vi "Servo MoveBy.vi"(8 "error in":errorcluster, 10 "Move by":dbl, 11 "Status in":T1={"Servo variables"={"Terget reached"=FALSE, "Connected"=FALSE, "Power ON"=FALSE, "Operation mode"=FALSE, "Actual position"=0.0, "Target position"=0.0}, "Servo constants"={"Name"=enum."AxisX", "Pos position limit [mm]"=0.0, "Neg position limit [mm]"=0.0, "Pos velocity limit"=0.0, "Neg velocity limit"=0.0, "Acceleration limit"=0.0}, "Connection"=variant}) -> (0 "error out":errorcluster, 1 "executed":bool, 2 "Target position":dbl, 3 "connection out":variant)   [LabVIEW 2024, in "Servo drive module.lvlib"]
doc: "Executes an additive move from an actual position to a desired position.\nParams:\nStatus in - actual status of servo drive.\nMove by - a numeric of desired change of position for servo drive.\nReturns: \nTrget position\nExecuted - True, if execution was sucessful."
uses:
  Servo drive module.lvlib
  ctl/Servo state.ctl
  ctl/Servo variables.ctl
  ctl/Servo constants.ctl
  ctl/Axis names.ctl
  <vilib>/Utility/error.llb/Error Cluster From Error Code.vi
  <vilib>/ErrorRing/Error Ring.xnode
  <vilib>/addons/eal4LabVIEW/eal4LabVIEW.lvlib
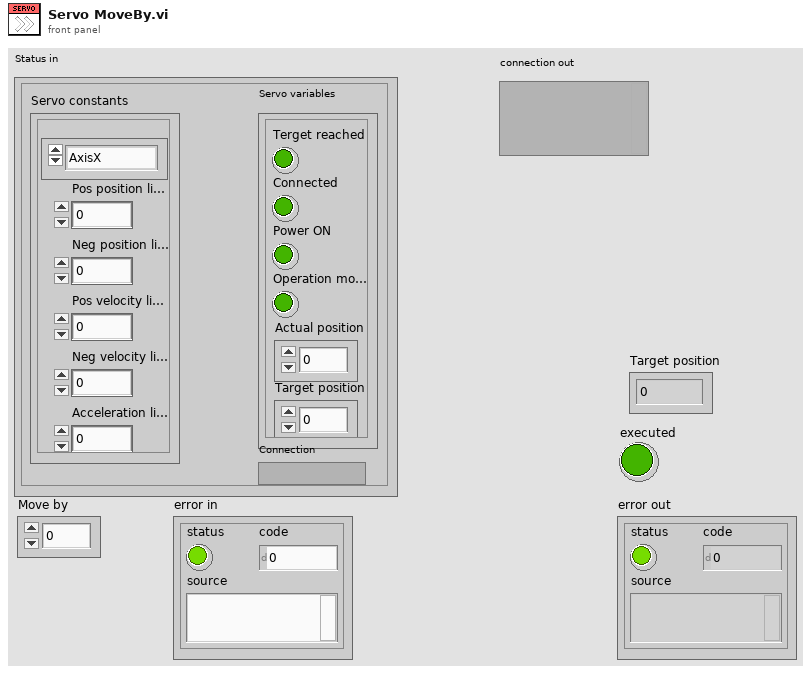
[diagram p1: front panel]
types:
  T1 = typedef "Servo drive module.lvlib/Servo state.ctl" = cluster{"Servo variables":T2, "Servo constants":T3, "Connection":variant}
  T2 = typedef "Servo drive module.lvlib/Servo variables.ctl" = cluster{"Terget reached":bool, "Connected":bool, "Power ON":bool, "Operation mode":bool, "Actual position":dbl, "Target position":dbl}
  T3 = typedef "Servo drive module.lvlib/Servo constants.ctl" = cluster{"Name":T4, "Pos position limit [mm]":dbl, "Neg position limit [mm]":dbl, "Pos velocity limit":dbl, "Neg velocity limit":dbl, "Acceleration limit":dbl}
  T4 = typedef "Servo drive module.lvlib/Axis names.ctl" = enum16{"Unknown", "AxisX", "AxisY", "AxisZ_left", "AxisZ_middle", "AxisZ_right"}
  T5 = cluster{"Position":dbl, "Velocity":dbl, "Acceleration":dbl, "Deceleration":dbl, "Jerk":dbl}
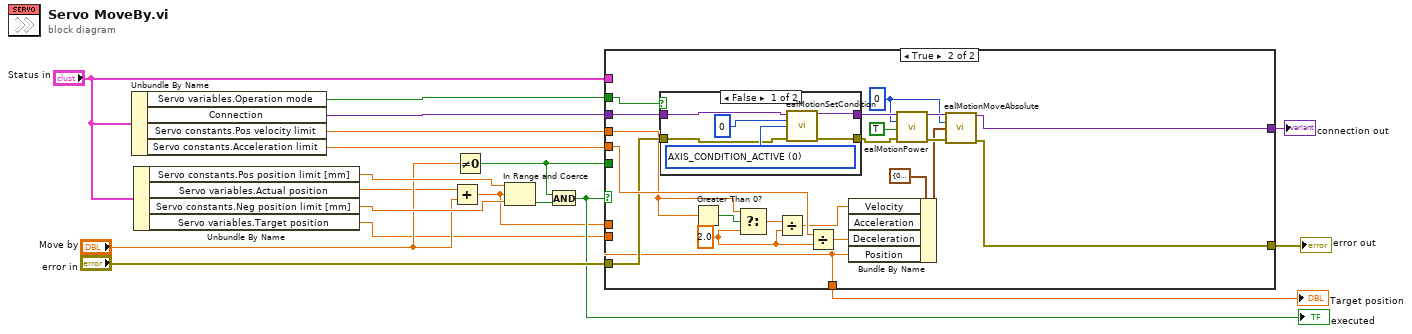
[diagram p0: block diagram]
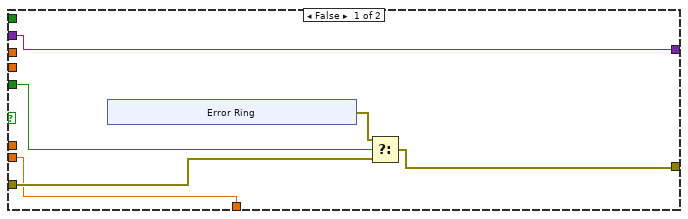
[diagram p2: hidden frame]
diagram:
  n1 = Unbundle By Name("Status in") -> ("Servo variables.Operation mode"=w16:bool, "Connection"=w15:variant, "Servo constants.Pos velocity limit"=w10:dbl, "Servo constants.Acceleration limit"=w9:dbl)
  n2 = Unbundle By Name("Status in") -> ("Servo constants.Pos position limit [mm]"=w14:dbl, "Servo variables.Actual position"=w2:dbl, "Servo constants.Neg position limit [mm]"=w13:dbl, "Servo variables.Target position"=w1:dbl)
  n3 = Add(x=w2, y="Move by") -> (x+y=w4:dbl)
  n4 = Not Equal To 0?(x="Move by") -> (x != 0?=w7:bool)
  n5 = In Range and Coerce(upper limit=w14, x=w4, lower limit=w13) -> (In Range?=w8:bool)  [unwired: 1 out]
  n6 = And(x=w7, y=w8) -> (x .and. y?=w5:bool)
  "executed" <- w5
  n7 = case shown="True" w5 {
    tunnel: w4 -> [_ w29]
    tunnel: [w24 w33] -> w18
    tunnel: "error in" -> [w22 w38]
    tunnel: "Status in" -> [_ _]
    tunnel: w15 -> [w20 w49]
    tunnel: w10 -> [_ w36]
    tunnel: w9 -> [_ w48]
    tunnel: w16 -> [_ w39]
    tunnel: w7 -> [w23 _]
    tunnel: [w20 w32] -> w6
    tunnel: [w19 w29] -> w3
    tunnel: w1 -> [w19 _]
    frame False {
      n8 = xnode "Error Ring"() -> ("error out"=w21:errorcluster)
      n9 = Select(t=w21, s=w23, f=w22) -> (s? t:f=w24:errorcluster)
    }
    frame True {
      w40 = 0 ("slave index")
      w34 = 2.0 ("y")
      n10 = case shown="False" w39 {
        tunnel: [w55 w57] -> w43
        tunnel: [w53 w56] -> w44
        tunnel: w49 -> [w52 w57]
        tunnel: w38 -> [w50 w56]
        frame False {
          w54 = 0 items=["AXIS_CONDITION_ACTIVE"=0, "AXIS_CONDITION_PARKING"=1, "AXIS_CONDITION_DEACTIVATED"=2, "AXIS_CONDITION_ACTIVE_DECOUPLED"=4, "AXIS_CONDITION_PARKING_DECOUPLED"=5, "AXIS_CONDITION_DEACTIVATED_DECOUPLED"=6, "AXIS_CONDITION_ACTIVE_PARAMETERIZATION"=8, "AXIS_CONDITION_PARKING_PARAMETERIZATION"=9, "AXIS_CONDITION_DEACTIVATED_PARAMETERIZATION"=10, "AXIS_CONDITION_ACTIVE_DECOUPLED_PARAMETERIZATION"=12, "AXIS_CONDITION_PARKING_DECOUPLED_PARAMETERIZATION"=13, "AXIS_CONDITION_DEACTIVATED_DECOUPLED_PARAMETERIZATION"=14] ("condition")
          n11 = call <vilib>:"ealMotionSetCondition.vi"("connection in"=w52, "slave index"=0, "condition"=w54, "error in (no error)"=w50) -> ("connection out"=w55:variant, "error out"=w53:errorcluster)  [unwired: 10 in]
        }
        frame True {
        }
      }
      n12 = Greater Than 0?(x=w36) -> (x > 0?=w37:bool)
      n13 = Select(t=w36, s=w37, f=w34) -> (s? t:f=w35:dbl)
      n14 = Divide(x=w35, y=w34) -> (x/y=w42:dbl)
      n15 = Divide(x=w48, y=w34) -> (x/y=w41:dbl)
      n16 = Bundle By Name(cluster=T5 {"Position"=0.0, "Velocity"=500.0, "Acceleration"=500.0, "Deceleration"=500.0, "Jerk"=500.0} ("parameter set"), "Velocity"=w42, "Acceleration"=w41, "Deceleration"=w41, "Position"=w29) -> (w31:T5)
      n17 = call <vilib>:"ealMotionPower.vi"("connection in"=w43, "slave index"=w40, "value"=TRUE, "error in (no error)"=w44) -> ("connection out"=w45:variant, "error out"=w46:errorcluster)  [unwired: 10 in]
      n18 = call <vilib>:"ealMotionMoveAbsolute.vi"("connection in"=w45, "slave index"=w40, "parameter set"=w31, "error in (no error)"=w46) -> ("connection out"=w32:variant, "error out"=w33:errorcluster)  [unwired: 10 in]
    }
  }
  "error out" <- w18
  "Target position" <- w3
  "connection out" <- w6
